vi "MSETNX.vi"(0 "TCP session out":refnum<k5>, 1 "Keys":string[](array[string]), 5 "Values":string[](array[string]), 11 "error in":errorcluster) -> (4 "TCP session out":refnum<k5>, 6 "Data":T1, 15 "error out":errorcluster)   [LabVIEW 2023]
uses:
  SubVIs/Controls/redis-data.ctl
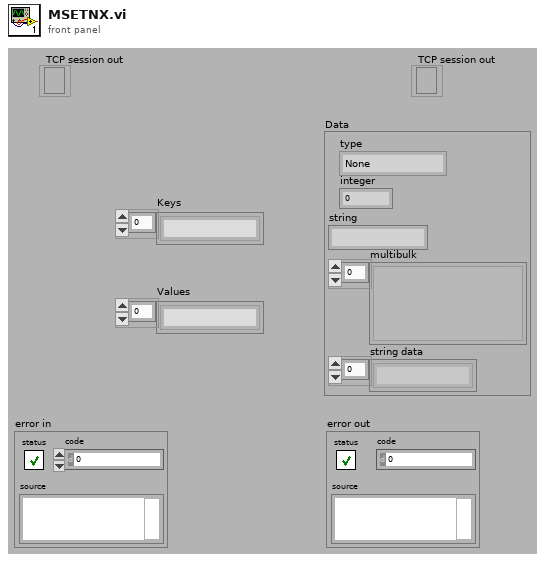
[diagram p1: front panel]
types:
  T1 = typedef "redis-data.ctl" = cluster{"type":enum16{"None", "Error", "Status", "Nil", "Integer", "String", "Multibulk"}, "integer":i64, "string":string, "multibulk":variant[], "string data":string[]}
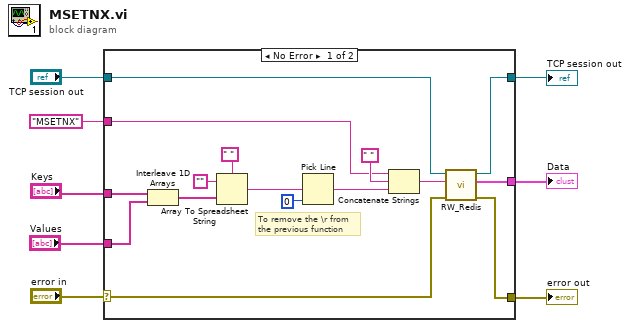
[diagram p0: block diagram]
diagram:
  n1 = case shown="No Error" "error in" {
    selector: "error in" -> [w16 w26]
    tunnel: "Keys" -> [w11 _]
    tunnel: "MSETNX" -> [w18 _]
    tunnel: "TCP session out" -> [w13 w25]
    tunnel: [w15 w26] -> w4
    tunnel: [w14 _] -> w3
    tunnel: [w9 w25] -> w2
    tunnel: "Values" -> [w12 _]
    frame No Error {
      # "To remove the \\r from\nthe previous function"
      n2 = Interleave 1D Arrays(w11, w12) -> (w10:string[])
      n3 = Array To Spreadsheet String(delimiter (Tab)=" ", array=w10, 3:"" ("format string")) -> (spreadsheet string=w20:string)
      n4 = Pick Line(multi-line string=w20, line index=0) -> (output string=w21:string)  [unwired: 1 in]
      n5 = Concatenate Strings(w18, " ", w21) -> (w17:string)
      n6 = call "RW_Redis.vi"("error in"=w16, "command"=w17, "TCP session in"=w13) -> ("error out"=w15:errorcluster, "Data"=w14:T1, "TCP session out"=w9:refnum<k5>)  [unwired: 6 in]
    }
    frame Error {
    }
  }
  "error out" <- w4
  "Data" <- w3
  "TCP session out" <- w2
